vi "Multi-mode acquisition.vi"() -> ()   [LabVIEW 2015]
doc: "Acquires sequences from the Andor iXon camera into Glimpse. \"Multi-mode\" means that the VI can be configured to sequentially acquire frames in multiple modes with different light sources and numbers of frames in each mode. Each mode is collected into a separate aquisition directory in Glimpse. Acquisition can be time-lapsed with a settable delay interval between cycles; the selected laser(s) are shuttered whilst not acquiring. The ixon setup acquisition.vi front panel is displayed so that the user can set the acquisition parameters before acquiring.\n\nThis is a Glimpse plug-in. To insure proper operation, you should have the source version of Glimpse running before loading this program. (The source version has an .llb extension, not a .exe one)."
uses:
  new-h-nu-ixon/Laser type.ctt
  new-h-nu-ixon/Emission filters.ctl
  ixon1024/HAL camera parameters important.ctt
  ixon1024/ixon readout settings.ctl
  ixon1024/andor acquisition mode.ctl
  Glimpse core/Video acquisition state.ctl
  <vilib>/vision/Image Controls.llb/IMAQ Image.ctl
  Glimpse core/Seq file v 1/Offset table.ctl
  Glimpse core/Seq file v 1/Offset.ctl
  Glimpse core/Seq file v 1/file number.ctl
  ixon1024/camera defaults globals.vi
  Stage/stage step to next field globals.vi
  Camera/camera globals.vi
  Glimpse core/GLIMPSE Globals.vi
  Autofocus Globals.vi
  new-h-nu-ixon/stage globals.vi
panel:
  in  "Max. number of acquisition files":i8(slide)=10 scale=0.0..50.0
  in  "Go? (F)":bool
  in  "Quit":bool
  in  "Delay after\nfilter change\n(ms)":u32
  in  "Scan fields options":T1(radio)
  in  "Scan Fields":bool
  in  "Max. cycles":i32=9999999
  in  "Cycle Interval (s)":dbl format="%_3f"
  in  "Camera Parameters":T2={"Exposure Time (sec)"=1.0, "EM CCD Gain"=230, "Readout Settings"={"Acquisition Mode"=enum."Frame Transfer Run till Abort", "Pixel Rate"=enum."EM CCD 5 Mhz 14 bits", "High Capacity?"=FALSE, "V Shift Speed (us/row)"=enum."6.5", "V Shift Amplitude"=enum."+1", "Preamp Gain"=enum."2.4", "Trigger Mode"=0, "Baseline offset"=0, "Baseline clamp"=TRUE}, "Image Size"={"H Bin"=1, "V Bin"=1, "Left"=1, "Top"=196, "Right"=1024, "Bottom"=730}} {"Readout Settings"."Baseline offset" min=-1000 max=1000 step=100; "Readout Settings"."Trigger Mode" items=["Internal", "External"]; "EM CCD Gain" scale=1.0..300.0; "Exposure Time (sec)" scale=0.001..10.0 scale format="%#_1g"}
  in  "Acquisition Protocol":T7(array[cluster]) {"Wait after frames (s)" format="%_3f"}
  # "Note:  In all panels, Ctrl-H displays the Context Help Window.  Hover mouse over panel icon or controls for context help."
  # "Camera: Andor iXon"
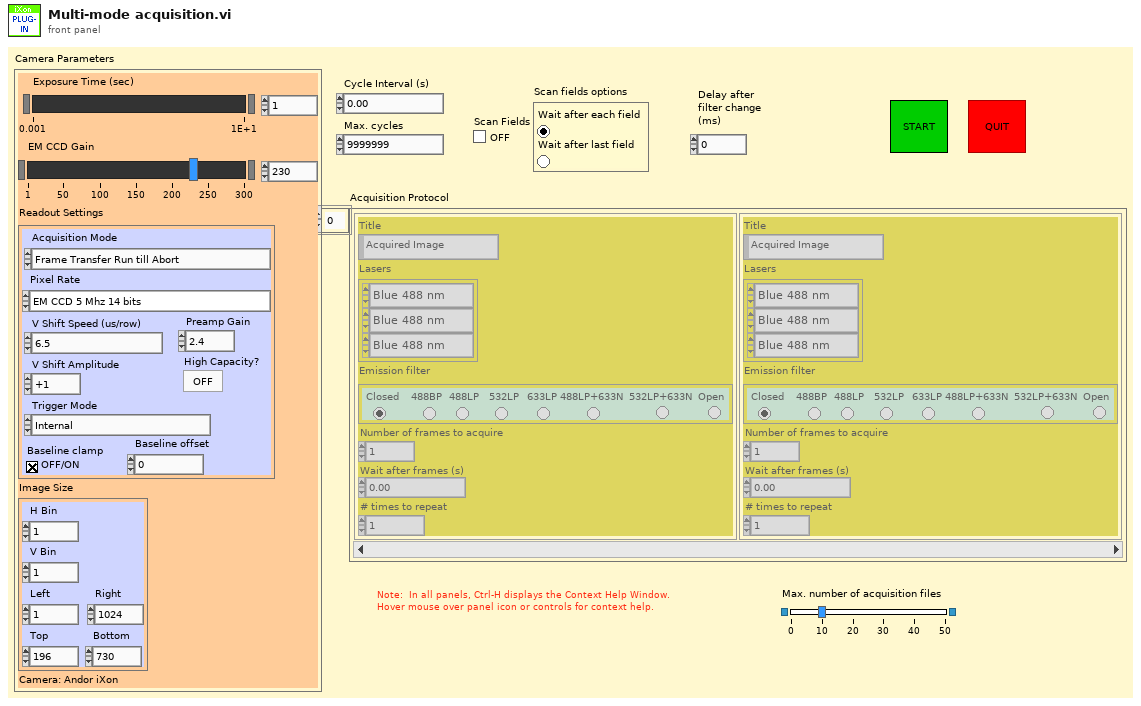
[diagram p1: front panel]
types:
  T1 = enum32{"Wait after each field", "Wait after last field"}
  T2 = typedef "HAL camera parameters important.ctt" = cluster{"Exposure Time (sec)":sgl, "EM CCD Gain":u16, "Readout Settings":T3, "Image Size":cluster{"H Bin":i32, "V Bin":i32, "Left":i32, "Top":i32, "Right":i32, "Bottom":i32}}
  T3 = typedef "ixon readout settings.ctl" = cluster{"Acquisition Mode":T4, "Pixel Rate":enum16{"EM CCD 10 Mhz 14 bits", "EM CCD 5 Mhz 14 bits", "EM CCD 3 Mhz 14 bits", "EM CCD 1 Mhz 16 bits", "Standard CCD 3 Mhz 14 bits", "Standard CCD 1 Mhz 16 bits"}, "High Capacity?":bool, "V Shift Speed (us/row)":enum16{"0.9 (not reccommended)", "1.7  (not reccommended)", "3.3  (not reccommended)", "6.5", "12.9"}, "V Shift Amplitude":enum16{"normal", "+1", "+2", "+3", "+4"}, "Preamp Gain":enum16{"1.0", "2.4", "5.0"}, "Trigger Mode":u32, "Baseline offset":i16, "Baseline clamp":bool}
  T4 = typedef "andor acquisition mode.ctl" = enum16{"(do not use)", "Single Scan", "Accumulate", "Kinetics", "Fast Kinetics", "Kinetics Run till Abort", "Frame Transfer", "Frame Transfer Run till Abort", "(do not use) ", "Time Delayed Integration"}
  T5 = typedef "Laser type.ctt" = enum16{"Blue 488 nm", "Green 532 nm", "Red 633 nm", "IR 780"}
  T6 = typedef "Emission filters.ctl" = enum32{" Closed ", " 488BP ", "488LP", "  532LP ", "633LP", "488LP+633N", "532LP+633N", "Open"}
  T7 = cluster{"Title":string, "Lasers":T5[], "Emission filter":T6, "Number of frames to acquire":i32, "Wait after frames (s)":dbl, "# times to repeat":i32}[]
  T8 = enum32{"None", "Manual", "Auto - Image analysis", "Auto - Retro-reflection"}
  T9 = typedef "image size.ctl" = cluster{"H Bin":i32, "V Bin":i32, "Left":i32, "Top":i32, "Right":i32, "Bottom":i32}
  T10 = typedef "Glimpse file parameters.ctt" = cluster{"Frame Size (bytes)":u32, "Max Frames":u32, "Max time (s)":u32, "Max Time (min)":u32, "Max Space Req'd. (Gb)":dbl, "Frames per acquisition file":u32}
  T11 = typedef "Video acquisition state.ctl" = cluster{"Pixel depth":enum32{"8 bits", "16 bits", "Float", "Complex", "RGB Chunky", "Compressed"}, "Width":dbl, "Height":dbl, "Buffer":T12, "Frames Acquired":u32, "Time of 1st frame":dbl, "TTB element zero":u32, "File Offsets Array":T13, "TTB Array":u32[], "Sum Image (for averaging)":T12, "Time at end of last acquisition (ms)":u32, "Filter array":u16[], "Flow rate array":dbl[], "Temperature array":dbl[], "Field array":u16[], "Lasers array":u16[][], "Stage xyz array":dbl[][]}
  T12 = typedef "IMAQ Image.ctl" = refnum<image>
  T13 = typedef "Offset table.ctl" = cluster{"offset":T14, "file number":T15}[]
  T14 = typedef "Offset.ctl" = i32
  T15 = typedef "file number.ctl" = u8
  T16 = typedef "Sequence files handle.ctt" = cluster{"Sequence files directory path":path, "Sequence files refnum array":refnum<file>[]}
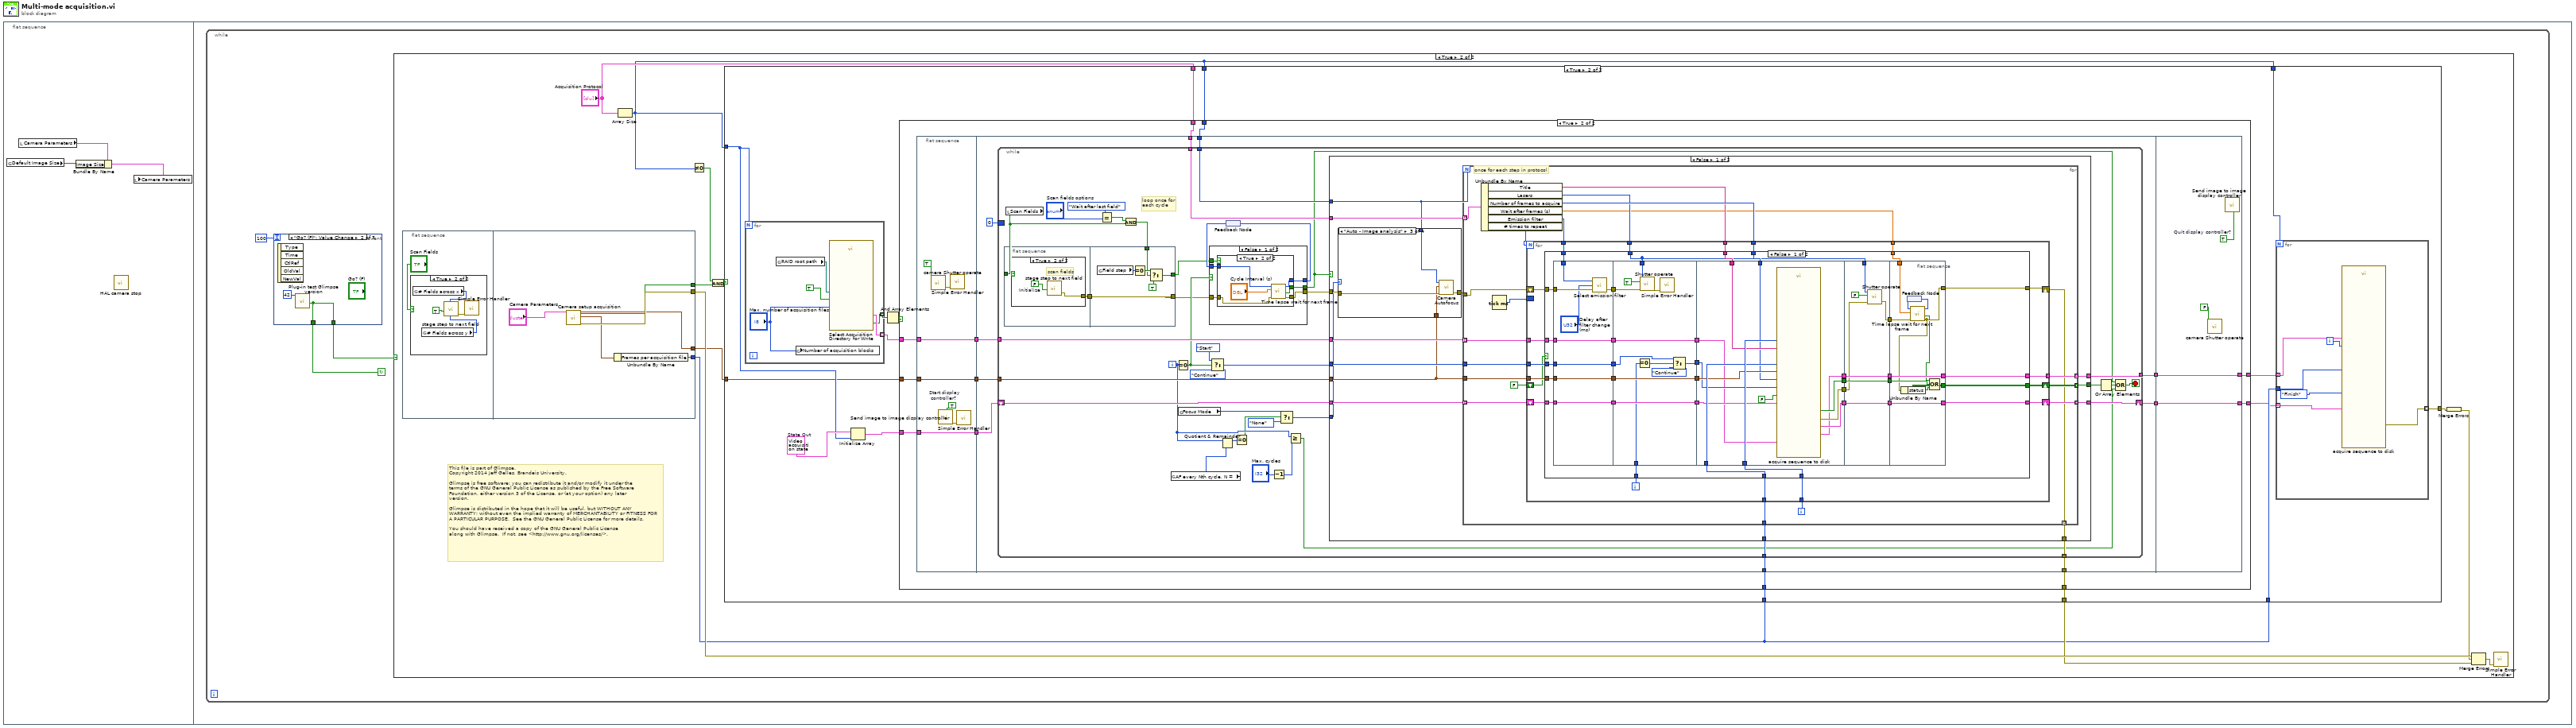
[diagram p0: block diagram]
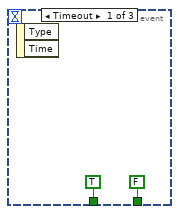
[diagram p2: hidden frame]
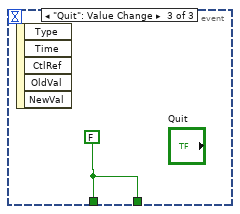
[diagram p3: hidden frame]
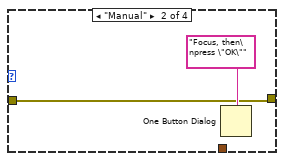
[diagram p9: hidden frame]
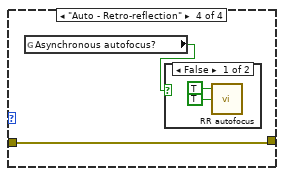
[diagram p10: hidden frame]
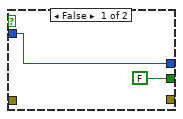
[diagram p15: hidden frame]
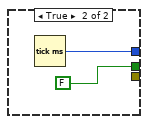
[diagram p16: hidden frame]
diagram:
  n1 = flat-sequence {
    frame #0 {
      n2 = global read "camera defaults globals.vi" "Default Image Size"() -> (w3:T9)
      n3 = local read "Camera Parameters"() -> (w2:T2)
      n4 = Bundle By Name(cluster=w2, "Image Size"=w3) -> (w1:T2)
      n5 = call "HAL camera stop.vi"() -> ()  [unwired: 1 in]
      n6 = local write "Camera Parameters"(w1) -> ()
    }
    frame #1 {
      n7 = while {
        stop <- w5 continue-if-true
        n8 = event shown="[1] \"Go? (F)\": Value Change" {
          selector: _ -> [_ _ _]
          dyn-events: _ -> [_ _ _]
          timeout: 100 -> [_ _ _]
          tunnel: [TRUE ("OK?") w9 w11] -> w5
          tunnel: [FALSE ("OK?") w9 w11] -> w4
          event Timeout {
            n9 = event-data() -> ()  [unwired: 1 in, 2 out]
          }
          event "Go? (F)": Value Change {
            n10 = event-data() -> ()  [unwired: 1 in, 5 out]
            n11 = call "Plug-in test Glimpse version.vi"("Minimum version required"=42) -> ("OK?"=w9:bool)  [unwired: 6 out]
          }
          event "Quit": Value Change {
            w11 = FALSE ("OK?")
            n12 = event-data() -> ()  [unwired: 1 in, 5 out]
          }
        }
        n13 = case shown="True" w4 {
          frame False {
          }
          frame True {
            # "This file is part of Glimpse. \nCopyright 2014 Jeff Gelles, Brandeis University.    \n\nGlimpse is free software: you can redistribute it and/or modify it under the \nterms of the GNU General Public License as published by the Free Software \nFoundation, either version 3 of the License, or (at your option) any later \nversion.\n\nGlimpse is distributed in the hope that it will be useful, but WITHOUT ANY \nWARRANTY; without even the implied warranty of MERCHANTABILITY or FITNESS FOR \nA PARTICULAR PURPOSE.  See the GNU General Public License for more details.\n\nYou should have received a copy of the GNU General Public License\nalong with Glimpse.  If not, see <http://www.gnu.org/licenses/>."
            n14 = flat-sequence {
              tunnel: [w34] -> w23
              tunnel: [w33] -> w17
              tunnel: [w32] -> w14
              tunnel: [w29] -> w12
              frame #0 {
                n15 = case shown="True" "Scan Fields" {
                  frame False {
                  }
                  frame True {
                    n16 = global read "stage step to next field globals.vi" "# Fields across x"() -> (w26:i8)
                    n17 = global read "stage step to next field globals.vi" "# Fields across y"() -> (w25:i8)
                    n18 = call "stage step to next field.vi"("# Fields across x"=w26, "Initialize"=TRUE, "# Fields across y"=w25) -> ("error out"=w28:errorcluster)  [unwired: 2 in, 3 out]
                    n19 = call <vilib>:"Simple Error Handler.vi"("error in (no error)"=w28) -> ()  [unwired: 1 in, 8 out]
                  }
                }
              }
              frame #1 {
                n20 = call "Camera setup acquisition.vi"("Camera Parameters (important)"="Camera Parameters") -> ("Image Size Out"=w32:T9, "Continue with acq?"=w33:bool, "Glimpse file properties"=w30:T10, "Error Out (no error)"=w34:errorcluster)  [unwired: 6 in, 9 out]
                n21 = Unbundle By Name(w30) -> ("Frames per acquisition file"=w29:u32)
              }
            }
            n22 = Array Size(array="Acquisition Protocol") -> (size(s)=w16:i32)
            n23 = Not Equal To 0?(x=w16) -> (x != 0?=w15:bool)
            n24 = And(x=w15, y=w17) -> (x .and. y?=w18:bool)
            n25 = case shown="True" w18 {
              tunnel: w12 -> [_ w49]
              tunnel: w12 -> [_ w48]
              tunnel: [_ w47] -> w21
              tunnel: [_ w46] -> w22
              tunnel: w16 -> [_ w36]
              tunnel: w16 -> [_ w42]
              tunnel: w16 -> [_ w39]
              tunnel: "Acquisition Protocol" -> [_ w37]
              tunnel: w14 -> [_ w35]
              frame False {
              }
              frame True {
                w41 = T11 {"Pixel depth"=enum."8 bits", "Width"=0.0, "Height"=0.0, "Buffer"=refnum, "Frames Acquired"=0, "Time of 1st frame"=0.0, "TTB element zero"=0, "File Offsets Array"=[], "TTB Array"=[], "Sum Image (for averaging)"=refnum, "Time at end of last acquisition (ms)"=0, "Filter array"=[], "Flow rate array"=[], "Temperature array"=[], "Field array"=[], "Lasers array"=[], "Stage xyz array"=[]}  # State Out
                n26 = for {
                  N: w36 -> [_]
                  tunnel: [w314] -> w38 mode=indexing
                  tunnel: [w313] -> w50 mode=indexing
                  n27 = global read "GLIMPSE Globals.vi" "RAID root path"() -> (w316:path)
                  n28 = global write "camera globals.vi" "Number of acquisition blocks"("Max. number of acquisition files") -> ()
                  n29 = call "Select Acquisition Directory for Write.vi"("Autostart?"=TRUE, "Acquisition directory root path"=w316, "Number of acquisition files"="Max. number of acquisition files") -> ("Sequence files handle"=w314:T16, "OK?"=w313:bool)  [unwired: 11 out]
                }
                n30 = Initialize Array(w41, w36) -> (w40:T11[])
                n31 = And Array Elements(Boolean array=w50) -> (logical AND=w43:bool)
                n32 = case shown="True" w43 {
                  tunnel: [w57 w72] -> w45
                  tunnel: w38 -> [w57 w71]
                  tunnel: w49 -> [_ w70]
                  tunnel: [w58 w69] -> w44
                  tunnel: [_ w68] -> w47
                  tunnel: w42 -> [_ w67]
                  tunnel: w40 -> [w58 w66]
                  tunnel: w37 -> [_ w65]
                  tunnel: w35 -> [_ w60]
                  frame False {
                  }
                  frame True {
                    n33 = flat-sequence {
                      tunnel: w66 -> [w78]
                      tunnel: w71 -> [w79]
                      tunnel: [w79] -> w64
                      tunnel: [w78] -> w63
                      tunnel: w60 -> [w76]
                      tunnel: [w76] -> w59
                      tunnel: w70 -> [w87]
                      tunnel: [w85] -> w68
                      tunnel: w67 -> [w84]
                      tunnel: w65 -> [w82]
                      tunnel: w64 -> [w88]
                      tunnel: w63 -> [w83]
                      tunnel: [w89] -> w62
                      tunnel: [w86] -> w61
                      tunnel: w59 -> [w81]
                      tunnel: [w310] -> w69
                      tunnel: [w311] -> w72
                      tunnel: w62 -> [w311]
                      tunnel: w61 -> [w310]
                      frame #0 {
                        w75 = TRUE  # Start display  controller?
                        n34 = call "camera Shutter operate.vi"("Open?"=TRUE) -> ("error out"=w73:errorcluster)  [unwired: 1 in, 6 out]
                        n35 = call "Send image to image display controller.vi"("Start display controller?"=w75) -> ("error out"=w74:errorcluster)  [unwired: 6 in, 3 out]
                        n36 = call <vilib>:"Simple Error Handler.vi"("error in (no error)"=w73) -> ()  [unwired: 1 in, 8 out]
                        n37 = call <vilib>:"Simple Error Handler.vi"("error in (no error)"=w74) -> ()  [unwired: 1 in, 8 out]
                      }
                      frame #1 {
                        n38 = while {
                          tunnel: [w127] -> w89
                          tunnel: w88 -> [w126]
                          tunnel: w87 -> [w125]
                          shift-right: [w123] -> w86
                          shift-left: w83 -> [w124]
                          tunnel: [w122] -> w85
                          tunnel: w84 -> [w110]
                          tunnel: w82 -> [w116]
                          tunnel: w81 -> [w111]
                          border: u32 0 -> [_]
                          i -> [w107]
                          stop <- w114 stop-if-true
                          # "loop once for\neach cycle"
                          n39 = flat-sequence {
                            tunnel: w96 -> [w283]
                            tunnel: [w282] -> w97
                            tunnel: [w291] -> w102
                            tunnel: w97 -> [w291]
                            tunnel: w94 -> [w287]
                            tunnel: [w286] -> w95
                            frame #0 {
                              n40 = case shown="True" w283 {
                                tunnel: [_ w284] -> w282
                                frame False {
                                }
                                frame True {
                                w285 = FALSE  # Initialize
                                # "scan fields"
                                n41 = call "stage step to next field.vi"("Initialize"=w285) -> ("error out"=w284:errorcluster)  [unwired: 4 in, 3 out]
                                }
                              }
                            }
                            frame #1 {
                              n42 = global read "stage globals.vi" "Field step"() -> (w288:i16)
                              n43 = Equal To 0?(x=w288) -> (x = 0?=w289:bool)
                              n44 = Select(t=w289, s=w287, f=TRUE) -> (s? t:f=w286:bool)
                            }
                          }
                          n45 = local read "Scan Fields"() -> (w96:bool)
                          n46 = Equal?(x="Scan fields options", y=T1."Wait after last field") -> (x = y?=w93:bool)
                          n47 = And(x=w93, y=w96) -> (x .and. y?=w94:bool)
                          n48 = global read "Autofocus Globals.vi" "AF every Nth cycle, N ="() -> (w109:u8)
                          n49 = Equal To 0?(x=w107) -> (x = 0?=w115:bool)
                          n50 = global read "Autofocus Globals.vi" "Focus Mode"() -> (w100:T8)
                          n51 = Select(t=enum16{"Start", "Continue", "Finish"}."Start" ("Operation"), s=w115, f=enum16{"Start", "Continue", "Finish"}."Continue" ("Operation")) -> (s? t:f=w119:enum16{"Start", "Continue", "Finish"})
                          n52 = Quotient & Remainder(x=w107, y=w109) -> (x-y*floor(x/y)=w108:i32)  [unwired: 1 out]
                          n53 = feedback #1() -> (w112:u32)
                          n54 = case shown="False" w115 {
                            tunnel: [w297 w307] -> w113
                            tunnel: [w296 FALSE] -> w90
                            tunnel: w112 -> [w295 _]
                            tunnel: [w294 _] -> w103
                            tunnel: w95 -> [w293 _]
                            tunnel: w102 -> [w292 _]
                            frame False {
                              n55 = case shown="True" w293 {
                                tunnel: [w299 w305] -> w297
                                tunnel: [FALSE ("Stopped?") w304] -> w296
                                tunnel: w295 -> [w299 w303]
                                tunnel: [_ w301] -> w294
                                tunnel: w292 -> [_ w300]
                                frame False {
                                }
                                frame True {
                                n56 = call "Time lapse wait for next frame.vi"("error in (no error)"=w300, "Frame Interval (s)"="Cycle Interval (s)", "Time of last frame in"=w303) -> ("error out"=w301:errorcluster, "Stopped?"=w304:bool, "Time of this frame out (ms)"=w305:u32)  [unwired: 4 out]
                                }
                              }
                            }
                            frame True {
                              n57 = Tick Count (ms)() -> (millisecond timer value=w307:u32)
                            }
                          }
                          n58 = feedback-in #1(w113) -> ()
                          n59 = Equal To 0?(x=w108) -> (x = 0?=w101:bool)
                          n60 = Decrement(x="Max. cycles") -> (x-1=w104:i32)
                          n61 = Select(t=w100, s=w101, f=T8."None") -> (s? t:f=w98:T8)
                          n62 = Greater Or Equal?(x=w107, y=w104) -> (x >= y?=w105:bool)
                          n63 = case shown="False" w90 {
                            tunnel: [w141 w280] -> w127
                            tunnel: w126 -> [w140 w280]
                            tunnel: w125 -> [w139 _]
                            tunnel: w124 -> [w138 w281]
                            tunnel: [w137 w281] -> w123
                            tunnel: [w136 _] -> w122
                            tunnel: w119 -> [w135 _]
                            tunnel: [w134 _] -> w118
                            tunnel: w116 -> [w133 _]
                            tunnel: w111 -> [w131 _]
                            tunnel: w110 -> [w130 _]
                            tunnel: w103 -> [w129 _]
                            tunnel: w98 -> [w128 _]
                            frame False {
                              n64 = case shown="\"Auto - Image analysis\"" w128 {
                                tunnel: w129 -> [w142 w143 w148 w150]
                                tunnel: [w142 w143 w147 w150] -> w132
                                tunnel: w131 -> [_ _ w146 _]
                                tunnel: w130 -> [_ _ w145 _]
                                frame "None", Default {
                                }
                                frame "Manual" {
                                n65 = One Button Dialog(message="Focus, then\npress \"OK\"") -> ()  [unwired: 2 out]
                                }
                                frame "Auto - Image analysis" {
                                n66 = call "Camera Autofocus.vi"("error in"=w148, "Image Size"=w146, "Display Window Number"=w145) -> ("error out"=w147:errorcluster)  [unwired: 2 in, 6 out]
                                }
                                frame "Auto - Retro-reflection" {
                                n67 = global read "Autofocus Globals.vi" "Asynchronous autofocus?"() -> (w149:bool)
                                n68 = case shown="False" w149 {
                                frame False {
                                n69 = call "RR autofocus.vi"("Close camera shutter during autofocus?"=TRUE, "Close laser shutter when autofocus is done?"=TRUE) -> ()  [unwired: 5 in, 1 out]
                                }
                                frame True {
                                }
                                }
                                }
                              }
                              n70 = for {
                                N: w130 -> [_]
                                tunnel: [w172] -> w141 mode=indexing
                                tunnel: w140 -> [w171] mode=indexing
                                tunnel: w139 -> [w170]
                                tunnel: w138 -> [w165] mode=indexing
                                tunnel: [w169] -> w137 mode=indexing
                                tunnel: [w168] -> w134 mode=indexing
                                tunnel: [w167] -> w136 mode=indexing
                                tunnel: w135 -> [w166]
                                tunnel: w133 -> [w164] mode=indexing
                                tunnel: w132 -> [w160]
                                tunnel: w131 -> [w159]
                                i -> [w162]
                                # "once for each step in protocol"
                                n71 = Unbundle By Name(w164) -> ("Title"=w161:string, "Lasers"=w158:T5[], "Number of frames to acquire"=w163:i32, "Wait after frames (s)"=w156:dbl, "Emission filter"=w153:T6, "# times to repeat"=w154:i32)
                                n72 = Tick Count (ms)() -> (millisecond timer value=w157:u32)
                                n73 = for {
                                N: w154 -> [_]
                                tunnel: [w190] -> w172
                                tunnel: w171 -> [w189]
                                tunnel: w170 -> [w188]
                                tunnel: w166 -> [w184]
                                tunnel: w163 -> [w182]
                                tunnel: w162 -> [w181]
                                tunnel: w161 -> [w180]
                                tunnel: w159 -> [w178]
                                tunnel: w158 -> [w177]
                                shift-right: [w187] -> w169
                                shift-left: w165 -> [w183]
                                border: w157 -> [_]
                                tunnel: w156 -> [w176]
                                shift-right: [w186] -> w168
                                shift-left: FALSE -> [w175]
                                shift-right: [w185] -> w167
                                shift-left: w160 -> [w179]
                                tunnel: w153 -> [w173]
                                i -> [w174]
                                n74 = case shown="False" w175 {
                                selector: w175 -> [_ w279]
                                tunnel: [w212 w276] -> w190
                                tunnel: w189 -> [w211 w276]
                                tunnel: w188 -> [w210 _]
                                tunnel: [w209 w278] -> w187
                                tunnel: [w208 w279] -> w186
                                tunnel: [w207 w277] -> w185
                                tunnel: w184 -> [w206 _]
                                tunnel: w183 -> [w205 w278]
                                tunnel: w182 -> [w204 _]
                                tunnel: w181 -> [w203 _]
                                tunnel: w180 -> [w202 _]
                                tunnel: w179 -> [w201 w277]
                                tunnel: w178 -> [w200 _]
                                tunnel: w177 -> [w199 _]
                                tunnel: w176 -> [w198 _]
                                tunnel: w174 -> [w197 _]
                                tunnel: w173 -> [w196 _]
                                frame False {
                                n75 = flat-sequence {
                                tunnel: w200 -> [w229]
                                tunnel: w201 -> [w227]
                                tunnel: w205 -> [w230]
                                tunnel: w206 -> [w231]
                                tunnel: w211 -> [w232]
                                tunnel: [w232] -> w195
                                tunnel: [w231] -> w194
                                tunnel: [w230] -> w193
                                tunnel: [w226] -> w192
                                tunnel: [w229] -> w191
                                tunnel: w196 -> [w228]
                                tunnel: [w244] -> w224
                                tunnel: w199 -> [w241]
                                tunnel: [w234] -> w223
                                tunnel: [w240] -> w222
                                tunnel: [w239] -> w221
                                tunnel: w197 -> [w236]
                                tunnel: w195 -> [w244]
                                tunnel: w194 -> [w235]
                                tunnel: w193 -> [w240]
                                tunnel: w192 -> [w233]
                                tunnel: w191 -> [w239]
                                tunnel: w224 -> [w246]
                                tunnel: [w247] -> w220
                                tunnel: [w245] -> w219
                                tunnel: [w248] -> w218
                                tunnel: w210 -> [w255]
                                tunnel: [w249] -> w217
                                tunnel: w223 -> [w252]
                                tunnel: w222 -> [w250]
                                tunnel: w204 -> [w253]
                                tunnel: w203 -> [w257]
                                tunnel: w202 -> [w256]
                                tunnel: w221 -> [w254]
                                tunnel: w220 -> [w264]
                                tunnel: [w264] -> w216
                                tunnel: w219 -> [w263]
                                tunnel: [w263] -> w215
                                tunnel: w218 -> [w259]
                                tunnel: w217 -> [w262]
                                tunnel: [w262] -> w214
                                tunnel: w199 -> [w260]
                                tunnel: [w258] -> w213
                                tunnel: [w274] -> w212
                                tunnel: [w275] -> w209
                                tunnel: w216 -> [w275]
                                tunnel: w215 -> [w274]
                                tunnel: w214 -> [w272]
                                tunnel: [w271] -> w208
                                tunnel: [w266] -> w207
                                tunnel: w198 -> [w268]
                                tunnel: w213 -> [w267]
                                frame #0 {
                                n76 = call "Select emission filter.vi"("Emission filter"=w228, "Time to wait\nafter filter change\n(ms)"="Delay after\nfilter change\n(ms)", "error in"=w227) -> ("error out"=w226:errorcluster)  [unwired: 3 out]
                                }
                                frame #1 {
                                n77 = Equal To 0?(x=w236) -> (x = 0?=w237:bool)
                                n78 = call "Shutter operate.vi"("Shutters"=w241, 2:TRUE ("Data to Write"), "error in"=w233) -> ("error out"=w242:errorcluster)  [unwired: 5 out]
                                n79 = call <vilib>:"Simple Error Handler.vi"("error in (no error)"=w242) -> ()  [unwired: 1 in, 8 out]
                                n80 = Select(t=w235, s=w237, f=enum16{"Start", "Continue", "Finish"}."Continue" ("Operation")) -> (s? t:f=w234:enum16{"Start", "Continue", "Finish"})
                                }
                                frame #2 {
                                n81 = call "acquire sequence to disk.vi"("Image Size"=w254, "State In"=w250, "Frames per acquisition file"=w255, "Sequence files handle"=w246, "Pressing stop automatically runs finish?"=FALSE, "Display Window Title"=w256, "Operation"=w252, "Display Window Number"=w257, "Number of frames to acquire"=w253) -> ("Done?"=w249:bool, "State Out"=w247:T11, "Sequence files handle out"=w245:T16, "error out"=w248:errorcluster)  [unwired: 2 in, 5 out]
                                }
                                frame #3 {
                                n82 = call "Shutter operate.vi"("Shutters"=w260, 2:FALSE ("Data to Write"), "error in"=w259) -> ("error out"=w258:errorcluster)  [unwired: 5 out]
                                }
                                frame #4 {
                                n83 = feedback #2() -> (w269:u32)
                                n84 = call "Time lapse wait for next frame.vi"("error in (no error)"=w267, "Frame Interval (s)"=w268, "Time of last frame in"=w269) -> ("error out"=w266:errorcluster, "Stopped?"=w265:bool, "Time of this frame out (ms)"=w270:u32)  [unwired: 4 out]
                                n85 = Unbundle By Name(w266) -> ("status"=w273:bool)
                                n86 = feedback-in #2(w270) -> ()
                                n87 = Compound Arithmetic op=OR(w265, w272, w273) -> (w271:bool)
                                }
                                }
                                }
                                frame True {
                                }
                                }
                                }
                              }
                            }
                            frame True {
                            }
                          }
                          n88 = Or Array Elements(Boolean array=w118) -> (logical OR=w117:bool)
                          n89 = Compound Arithmetic op=OR(w90, w117, w105) -> (w114:bool)
                        }
                      }
                      frame #2 {
                        w309 = TRUE  # Quit display controller?
                        n90 = call "camera Shutter operate.vi"("Open?"=FALSE) -> ()  [unwired: 1 in, 7 out]
                        n91 = call "Send image to image display controller.vi"("Quit display controller?"=w309) -> ()  [unwired: 6 in, 4 out]
                      }
                    }
                  }
                }
                n92 = for {
                  N: w39 -> [_]
                  tunnel: w48 -> [w54]
                  tunnel: [w51] -> w46 mode=indexing
                  tunnel: w45 -> [w56] mode=indexing
                  tunnel: w44 -> [w52] mode=indexing
                  i -> [w55]
                  n93 = call "acquire sequence to disk.vi"("State In"=w52, "Frames per acquisition file"=w54, "Sequence files handle"=w56, "Operation"=enum16{"Start", "Continue", "Finish"}."Finish", "Display Window Number"=w55) -> ("error out"=w51:errorcluster)  [unwired: 6 in, 8 out]
                }
              }
            }
            n94 = Merge Errors(w22) -> (w20:errorcluster)
            n95 = Merge Errors(w23, w20, w21) -> (w13:errorcluster)
            n96 = call <vilib>:"Simple Error Handler.vi"("error in (no error)"=w13) -> ()  [unwired: 1 in, 8 out]
          }
        }
      }
    }
  }
